vi "HT3_Finish.vi"(5 "FileHeaderPos":T1, 6 "Rates":dbl[](array[numeric]), 7 "Stop Reason":enum16{"timeover", "manual", "overflow"}(ring), 8 "error in":errorcluster, 9 "Num Records":i64, 10 "Stop After (ms)":i32, 11 "refnum in":refnum<file>) -> (0 "error out":errorcluster)   [LabVIEW 2009]
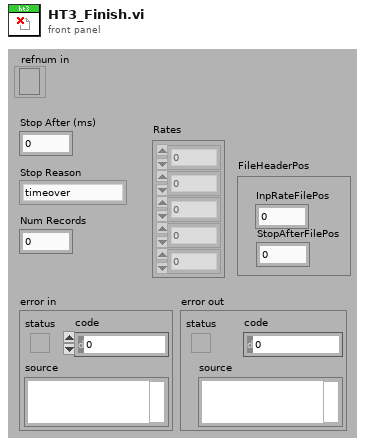
[diagram p1: front panel]
types:
  T1 = cluster{"InpRateFilePos":i64, "StopAfterFilePos":i64}
  T2 = enum16{"big-endian, network order", "native, host order", "little-endian"}
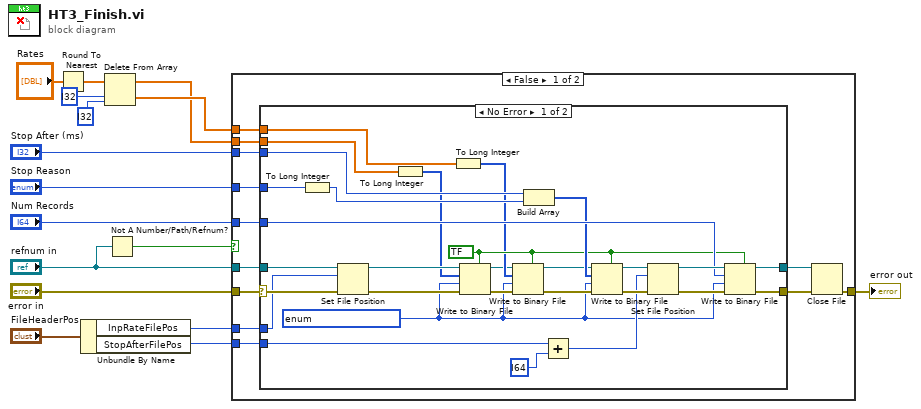
[diagram p0: block diagram]
diagram:
  n1 = Round To Nearest(number="Rates") -> (nearest integer value=w1:dbl[])
  n2 = Unbundle By Name("FileHeaderPos") -> ("InpRateFilePos"=w8:i64, "StopAfterFilePos"=w7:i64)
  n3 = Delete From Array(array=w1, length=i32 ?, index=i32 ?) -> (deleted portion=w4:dbl[], array with subset deleted=w3:dbl[])
  n4 = Not A Number/Path/Refnum?(number/path/refnum="refnum in") -> (NaN/Path/Refnum?=w11:bool)
  n5 = case shown="False" w11 {
    tunnel: "error in" -> [w28 w60]
    tunnel: "refnum in" -> [w27 _]
    tunnel: [w26 w60] -> w15
    tunnel: "Stop Reason" -> [w23 _]
    tunnel: "Num Records" -> [w22 _]
    tunnel: "Stop After (ms)" -> [w21 _]
    tunnel: w3 -> [w20 _]
    tunnel: w4 -> [w19 _]
    tunnel: w8 -> [w18 _]
    tunnel: w7 -> [w17 _]
    frame #0 {
      n6 = case shown="No Error" w28 {
        selector: w28 -> [w57 w58]
        tunnel: w27 -> [w56 w59]
        tunnel: [w47 w58] -> w25
        tunnel: [w44 w59] -> w24
        tunnel: w23 -> [w53 _]
        tunnel: w22 -> [w43 _]
        tunnel: w21 -> [w51 _]
        tunnel: w20 -> [w34 _]
        tunnel: w19 -> [w31 _]
        tunnel: w18 -> [w52 _]
        tunnel: w17 -> [w41 _]
        frame #0 {
          w35 = T2 ? ("byte order (0:big-endian, network order)")
          w36 = bool ? ("prepend array or string size? (T)")
          n7 = To Long Integer(number=w53) -> (32bit integer=w50:i32)
          n8 = Set File Position(offset (in bytes) (0)=w52, refnum=w56, error in=w57) -> (refnum out=w54:refnum<file>, error out=w55:errorcluster)  [unwired: 1 out]
          n9 = To Long Integer(number=w34) -> (32bit integer=w32:i32[])
          n10 = To Long Integer(number=w31) -> (32bit integer=w33:i32[])
          n11 = Write to Binary File(file (use dialog)=w54, data=w32, error in=w55, 5:w36, 9:w35) -> (refnum out=w29:refnum<file>, error out=w38:errorcluster)  [unwired: 2 out]
          n12 = Write to Binary File(file (use dialog)=w29, data=w33, error in=w38, 5:w36, 9:w35) -> (refnum out=w30:refnum<file>, error out=w37:errorcluster)  [unwired: 1 in, 1 out]
          n13 = Build Array(w51, w50) -> (w42:i32[])
          n14 = Add(x=w41, y=i64 ?) -> (x+y=w39:i64)
          n15 = Write to Binary File(file (use dialog)=w30, data=w42, error in=w37, 5:w36, 9:w35) -> (refnum out=w46:refnum<file>, error out=w49:errorcluster)  [unwired: 2 out]
          n16 = Set File Position(offset (in bytes) (0)=w39, refnum=w46, error in=w49) -> (refnum out=w45:refnum<file>, error out=w48:errorcluster)  [unwired: 1 out]
          n17 = Write to Binary File(file (use dialog)=w45, data=w43, error in=w48, 5:w36, 9:w35) -> (refnum out=w44:refnum<file>, error out=w47:errorcluster)  [unwired: 2 out]
        }
        frame #1 {
        }
      }
      n18 = Close File(refnum=w24, error in=w25) -> (error out=w26:errorcluster)  [unwired: 1 out]
    }
    frame #1 {
    }
  }
  "error out" <- w15
